vi "Handle Response to Client.vi"(10 "Response":T1, 11 "Session in":refnum<class "Session.lvclass">) -> (0 "error out":errorcluster)   [LabVIEW 2013, in "MQTT Server.lvlib" / "Session.lvclass"]
uses:
  Session.lvclass
  Server class/Response -- cluster.ctl
  Control Packets/ControlPacket/ControlPacket.lvclass
  Session.lvclass/Session.ctl
  Connection/TCPConnection.lvclass
  Server class/Server.lvclass
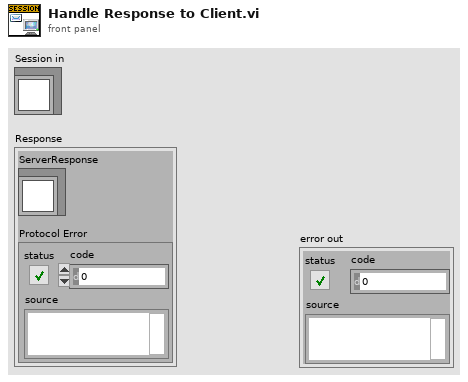
[diagram p1: front panel]
types:
  T1 = typedef "MQTT Server.lvlib/Server.lvclass/Response -- cluster.ctl" = cluster{"ServerResponse":refnum<class "ControlPacket.lvclass">, "Protocol Error":errorcluster}
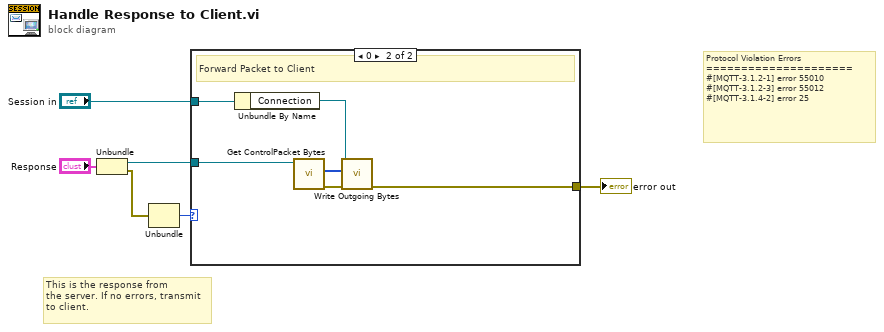
[diagram p0: block diagram]
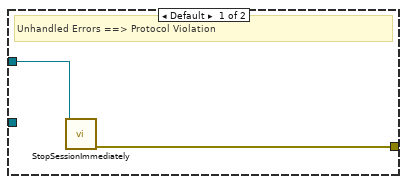
[diagram p2: hidden frame]
diagram:
  # "This is the response from\nthe server. If no errors, transmit\nto client."
  # "Protocol Violation Errors\n=====================\n#[MQTT-3.1.2-1] error 55010\n#[MQTT-3.1.2-3] error 55012\n#[MQTT-3.1.4-2] error 25"
  n1 = Unbundle("Response") -> ("ServerResponse"=w6:refnum<class "ControlPacket.lvclass">, "Protocol Error"=w1:errorcluster)
  n2 = Unbundle(w1) -> ("code"=w4:i32)  [unwired: 2 out]
  n3 = case shown="0" w4 {
    tunnel: w6 -> [_ w13]
    tunnel: [w8 w11] -> w3
    tunnel: "Session in" -> [w7 w10]
    frame Default {
      # "Unhandled Errors ==> Protocol Violation"
      n4 = call "StopSessionImmediately.vi"("Session in"=w7) -> ("error out"=w8:errorcluster)  [unwired: 9 in, 1 out]
    }
    frame 0 {
      # "Forward Packet to Client"
      n5 = Unbundle By Name(w10) -> ("Connection"=w9:refnum<class "TCPConnection.lvclass">)
      n6 = call "Get ControlPacket Bytes.vi"("ControlPacket"=w13) -> ("error out"=w12:errorcluster, "Bytes Stream"=w14:u8[])  [unwired: 8 in, 1 out]
      n7 = call "Write Outgoing Bytes.vi"("error in (no error)"=w12, "Bytes"=w14, "TCPConnection in"=w9) -> ("error out"=w11:errorcluster)  [unwired: 7 in, 1 out]
    }
  }
  "error out" <- w3
